vi "LidarTester.vi"() -> ()   [LabVIEW 2024]
uses:
  e33ea129-5426-40bd-9da2-e127971607b1.vi
  <vilib>/Instr/_visa.llb/VISA Configure Serial Port (Instr).vi
panel:
  in  "Tab Control":enum32{"Lidar", "Buffer"}(tab)
  out "LiDAR_ROI":cluster{i32[], i32[]}(graph)
  in  "COM4 2":refnum<visa-resource-name>="COM3" caption="LiDAR_Com."
  in  "격자크기":dbl=20.0
  in  "Stop":bool
  out "Loop Time":u32=102
  out "read buffer":string
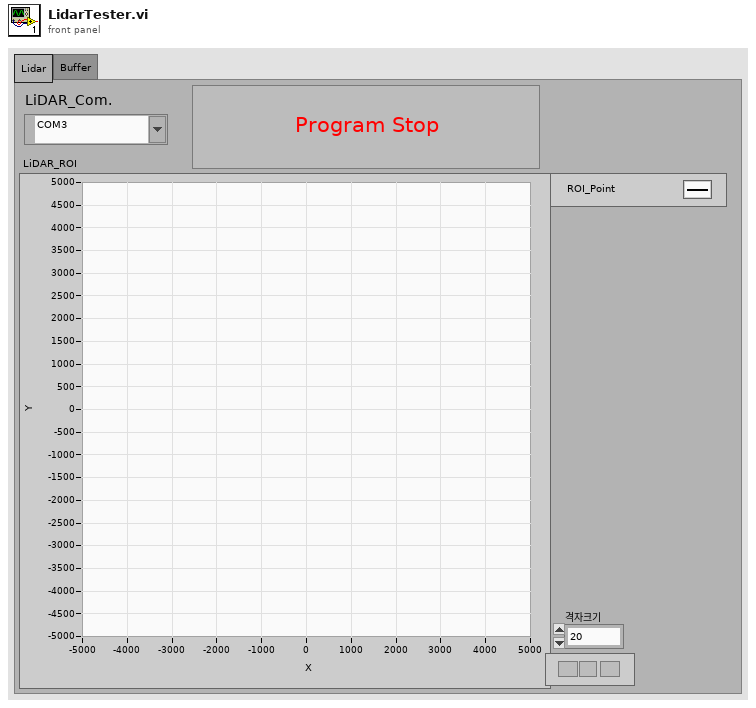
[diagram p1: front panel]
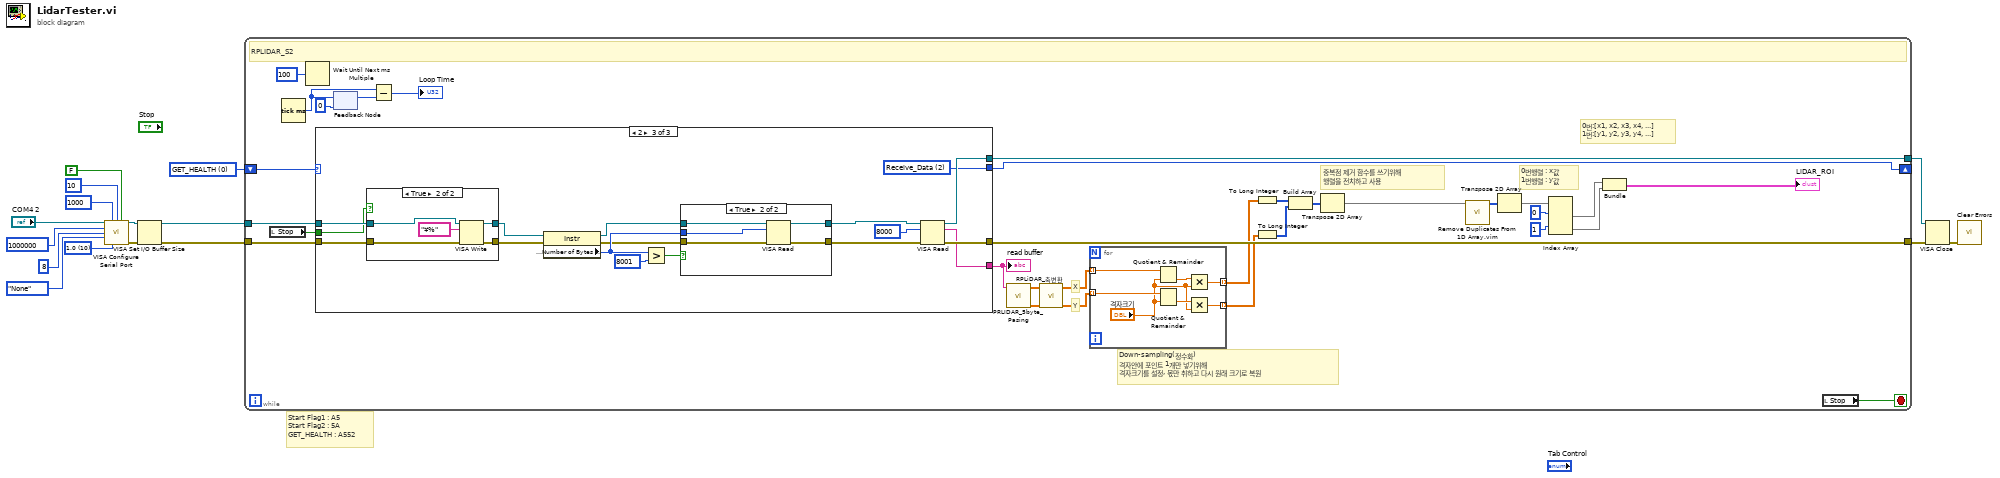
[diagram p0: block diagram]
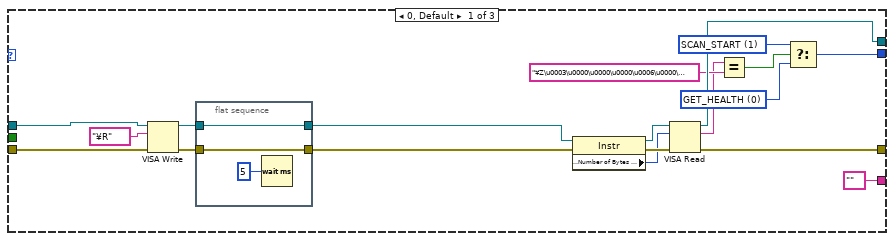
[diagram p2: hidden frame]
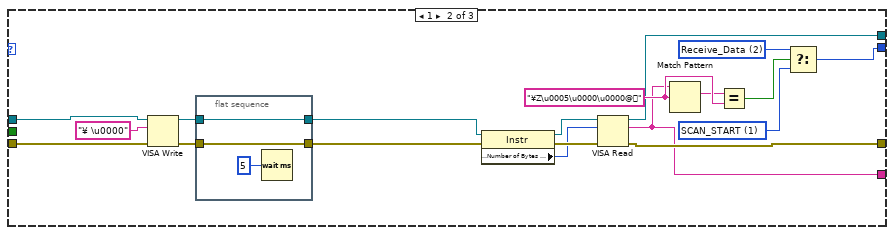
[diagram p3: hidden frame]
diagram:
  w1 = u16 10 items=["1.0"=10, "1.5"=15, "2.0"=20] ("stop bits (10: 1 bit)")
  w3 = u16 0 items=["GET_HEALTH", "SCAN_START", "Receive_Data"]
  # "Start Flag1 : A5\nStart Flag2 : 5A \nGET_HEALTH : A552"
  n1 = call-poly "VISA Configure Serial Port"("VISA resource name"="COM4 2", "timeout (10sec)"=u32 1000, "termination char\n(0xA = '\\n' = LF)"=u8 10 ("termination char\n(0xA = '\\n' = LF)"), "Enable Termination\nChar (T)"=FALSE ("Enable Termination\nChar (T)"), "baud rate (9600)"=u32 1000000, "data bits (8)"=u16 8, "parity (0:none)"=enum16{"None", "Odd", "Even", "Mark", "Space"}."None", "stop bits (10: 1 bit)"=w1) -> ("VISA resource name out"=w11:refnum<visa-resource-name>, "error out"=w10:errorcluster)  [unwired: 6 in]
  n2 = VISA Set I/O Buffer Size(VISA resource name=w11, error in (no error)=w10) -> (VISA resource name out=w5:refnum<visa-resource-name>, error out=w4:errorcluster)  [unwired: 2 in]
  n3 = while {
    tunnel: [w37] -> w15
    tunnel: [w38] -> w14
    tunnel: w5 -> [w46]
    tunnel: w4 -> [w45]
    shift-right: [w44] -> _
    shift-left: w3 -> [w47]
    stop <- w20 stop-if-true
    # "0번:[x1, x2, x3, x4, ...]\n1번:[y1, y2, y3, y4, ...]"
    # "0번행렬 : x값\n1번행렬 : y값"
    # "중복점 제거 함수를 쓰기위해\n행렬을 전치하고 사용"
    # "Down-sampling(정수화)\n격자안에 포인트 1개만 넣기위해\n격자크기를 설정, 몫만 취하고 다시 원래 크기로 복원"
    # "Y"
    # "X"
    # "RPLIDAR_S2"
    n4 = local read "Stop"() -> (w43:bool)
    n5 = Tick Count (ms)() -> (millisecond timer value=w42:u32)
    n6 = Wait Until Next ms Multiple(millisecond multiple=u32 100 ("ms 배수")) -> ()  [unwired: 1 out]
    n7 = case shown="2" w47 {
      tunnel: w46 -> [w72 w90 w113]
      tunnel: w45 -> [w71 w89 w112]
      tunnel: [w73 w86 w99] -> w44
      tunnel: [w62 w87 w115] -> w38
      tunnel: [w61 w88 w114] -> w37
      tunnel: w43 -> [_ _ w111]
      tunnel: ["" ("read buffer") w84 w110] -> w21
      frame 0, Default {
        w55 = u16 0 items=["GET_HEALTH", "SCAN_START", "Receive_Data"]
        w56 = u16 1 items=["GET_HEALTH", "SCAN_START", "Receive_Data"]
        n8 = VISA Write(VISA resource name=w72, write buffer="¥R", error in (no error)=w71) -> (VISA resource name out=w66:refnum<visa-resource-name>, error out=w65:errorcluster)  [unwired: 1 out]
        n9 = flat-sequence {
          tunnel: w66 -> [w75]
          tunnel: w65 -> [w74]
          tunnel: [w75] -> w64
          tunnel: [w74] -> w63
          frame #0 {
            n10 = Wait (ms)(milliseconds to wait=u32 5 ("대기 시간 (ms)")) -> ()  [unwired: 1 out]
          }
        }
        n11 = property class="Instr"(reference=w64, error in=w63) -> (reference out=w69:refnum<visa-resource-name>, error out=w68:errorcluster, "Serial Settings:Number of Bytes at Serial Port"=w67:u32)
        n12 = VISA Read(VISA resource name=w69, byte count=w67, error in (no error)=w68) -> (VISA resource name out=w61:refnum<visa-resource-name>, read buffer=w58:string, error out=w62:errorcluster)  [unwired: 1 out]
        n13 = Equal?(x=w58, y="¥Z\u0003\u0000\u0000\u0000\u0006\u0000\u0000\u0000") -> (x = y?=w59:bool)
        n14 = Select(t=w56, s=w59, f=w55) -> (s? t:f=w73:u16)
      }
      frame 1 {
        w77 = u16 2 items=["GET_HEALTH", "SCAN_START", "Receive_Data"]
        w78 = u16 1 items=["GET_HEALTH", "SCAN_START", "Receive_Data"]
        w91 = "¥Z\u0005\u0000\u0000@"
        n15 = VISA Write(VISA resource name=w90, write buffer="¥ \u0000", error in (no error)=w89) -> (VISA resource name out=w93:refnum<visa-resource-name>, error out=w94:errorcluster)  [unwired: 1 out]
        n16 = flat-sequence {
          tunnel: w93 -> [w97]
          tunnel: w94 -> [w96]
          tunnel: [w97] -> w80
          tunnel: [w96] -> w79
          frame #0 {
            n17 = Wait (ms)(milliseconds to wait=u32 5 ("대기 시간 (ms)")) -> ()  [unwired: 1 out]
          }
        }
        n18 = property class="Instr"(reference=w80, error in=w79) -> (reference out=w83:refnum<visa-resource-name>, error out=w82:errorcluster, "Serial Settings:Number of Bytes at Serial Port"=w81:u32)
        n19 = VISA Read(VISA resource name=w83, byte count=w81, error in (no error)=w82) -> (VISA resource name out=w88:refnum<visa-resource-name>, read buffer=w84:string, error out=w87:errorcluster)  [unwired: 1 out]
        n20 = Match Pattern(string=w84, regular expression=w91) -> (match substring=w85:string)  [unwired: 1 in, 3 out]
        n21 = Equal?(x=w85, y=w91) -> (x = y?=w95:bool)
        n22 = Select(t=w77, s=w95, f=w78) -> (s? t:f=w86:u16)
      }
      frame 2 {
        w99 = u16 2 items=["GET_HEALTH", "SCAN_START", "Receive_Data"]
        n23 = case shown="True" w111 {
          tunnel: w113 -> [w124 w128]
          tunnel: w112 -> [w123 w127]
          tunnel: [w124 w126] -> w109
          tunnel: [w123 w125] -> w108
          frame False {
          }
          frame True {
            n24 = VISA Write(VISA resource name=w128, write buffer="¥%", error in (no error)=w127) -> (VISA resource name out=w126:refnum<visa-resource-name>, error out=w125:errorcluster)  [unwired: 1 out]
          }
        }
        n25 = property class="Instr"(reference=w109, error in=w108) -> (reference out=w104:refnum<visa-resource-name>, error out=w103:errorcluster, "Serial Settings:Number of Bytes at Serial Port"=w105:u32)
        n26 = Greater?(x=w105, y=u32 8001) -> (0:w107:bool)
        n27 = case shown="True" w107 {
          tunnel: w104 -> [w117 w122]
          tunnel: w105 -> [_ w121]
          tunnel: w103 -> [w116 w120]
          tunnel: [w117 w119] -> w102
          tunnel: [w116 w118] -> w101
          frame False {
          }
          frame True {
            n28 = VISA Read(VISA resource name=w122, byte count=w121, error in (no error)=w120) -> (VISA resource name out=w119:refnum<visa-resource-name>, error out=w118:errorcluster)  [unwired: 2 out]
          }
        }
        n29 = VISA Read(VISA resource name=w102, byte count=u32 8000, error in (no error)=w101) -> (VISA resource name out=w114:refnum<visa-resource-name>, read buffer=w110:string, error out=w115:errorcluster)  [unwired: 1 out]
      }
    }
    "read buffer" <- w21
    n30 = feedback #1(u32 0 ("millisecond timer value")) -> (w41:u32)
    n31 = feedback-in #1(w42) -> ()
    n32 = Subtract(x=w42, y=w41) -> (x-y=→"Loop Time":u32)
    n33 = call "PRLIDAR_5byte_Pasing.vi"("RPLIDAR_Data"=w21) -> ("Theta(deg)"=w24:dbl[], "Distance(mm)"=w25:dbl[])  [unwired: 9 in]
    n34 = call "RPLiDAR_축변환.vi"("Distance(mm)"=w24, "Theta(deg)"=w25) -> ("Y"=w22:dbl[], "X"=w23:dbl[])  [unwired: 8 in]
    n35 = for {
      tunnel: w23 -> [w54] mode=indexing
      tunnel: w22 -> [w53] mode=indexing
      tunnel: [w50] -> w35 mode=indexing
      tunnel: [w49] -> w36 mode=indexing
      n36 = Quotient & Remainder(x=w54, y="격자크기") -> (floor(x/y)=w52:dbl)  [unwired: 1 out]
      n37 = Quotient & Remainder(x=w53, y="격자크기") -> (floor(x/y)=w51:dbl)  [unwired: 1 out]
      n38 = Multiply(x=w52, y="격자크기") -> (x*y=w50:dbl)
      n39 = Multiply(x=w51, y="격자크기") -> (x*y=w49:dbl)
    }
    n40 = To Long Integer(number=w35) -> (32bit integer=w29:i32[])
    n41 = To Long Integer(number=w36) -> (32bit integer=w28:i32[])
    n42 = Build Array(w29, w28) -> (w31:i32[][])
    n43 = Transpose 2D Array(2D array=w31) -> (transposed array=w26:i32[][])
    n44 = call "Remove Duplicates From 1D Array.vim"("array"=w26) -> ("array with duplicates removed"=w27:i32[][])  [unwired: 10 in]
    n45 = Transpose 2D Array(2D array=w27) -> (transposed array=w32:i32[][])
    n46 = Index Array(array=w32, index (row) #1=0 ("index (row)"), index (row) #2=1 ("index (row)")) -> (element #1=w19:i32[], element #2=w18:i32[])  [unwired: 2 in]
    n47 = Bundle(w19, w18) -> (→"LiDAR_ROI":cluster{i32[], i32[]})  [unwired: 1 in]
    n48 = local read "Stop"() -> (w20:bool)
  }
  n49 = VISA Close(VISA resource name=w15, error in (no error)=w14) -> (error out=w16:errorcluster)
  n50 = call <vilib>:"Clear Errors.vi"("error in (no error)"=w16) -> ()  [unwired: 5 in, 2 out]
